vi "niFpga wdp fft input buffer.vi"(4 "enable":bool, 6 "write memory 2?":bool, 8 "read index":fxp<+,9,9>, 9 "write index":fxp<+,8,8>, 10 "data in im":fxp<+/-,8,1>[](array[numeric])=[0.0, 0.0], 11 "data in re":fxp<+/-,8,1>[](array[numeric])=[0.0, 0.0]) -> (2 "data out 1":T1, 3 "data out 0":T1)   [LabVIEW 2017]
uses:
  <vilib>/rvi/Analysis/measure/FFT/config/niFpgaFFTIOPattern.ctl
  <vilib>/rvi/Emulation/niFpgaSctlEmulationGetInTimedLoop.vi
  <vilib>/Utility/error.llb/Clear Errors.vi
  <vilib>/rvi/DataTransferAndStorage/Container/Common/niFpgaContainerGetUniqueNameForEmu.vi
  <vilib>/rvi/DataTransferAndStorage/Container/Common/niFpgaContainerSetEmuInfo.vi
  <vilib>/rvi/eio/common/nirviEmuReportErrorAndStop.vi
  <vilib>/rvi/DataTransferAndStorage/Container/Common/niFpgaContainerExecOnDevCompGetState.vi
  <vilib>/rvi/Emulation/niFpgaEmulationIsFPGAContextNoSignature.vi
  <vilib>/rvi/Emulation/niFpgaProcessEmulError.vi
  <vilib>/rvi/errors/nirviReportUnexpectedCaseInternalError (U32).vi
  <vilib>/rvi/Memory/Memory_Emulation/niFpgaMemoryEmulationCacheClearOnFirstRun.vi
  <vilib>/rvi/Memory/Memory_Emulation/nirvimemoryEmulationManagerCache_MakeExclusive.vi
  <vilib>/rvi/Memory/Memory_Emulation/niFpgaMemoryEmulationValidateCache.vi
  <vilib>/rvi/Memory/Memory_Emulation/nirvimemoryEmulationManagerCache_InsertValue.vi
  <vilib>/rvi/Memory/Memory_Emulation/nirvimemoryEmulationManagerCache_ReleaseExclusive.vi
  <vilib>/rvi/Memory/Memory_Emulation/nirvimemoryEmulationManagerCache_GetValue.vi
  <vilib>/rvi/Memory/Memory_Emulation/nirvimemoryEmulationManagerCache_SetValue.vi
  <vilib>/rvi/Emulation/niFpgaSctlEmulationResourceMgr.vi
  <vilib>/rvi/LocalResourceManager/LocalResourceManager.xnode
  <vilib>/rvi/DataTransferAndStorage/Container/XNode/niFpgaContainer.xnode
  <vilib>/rvi/Memory/Memory_Emulation/niFpgaMemoryEmulationRefIn.vi
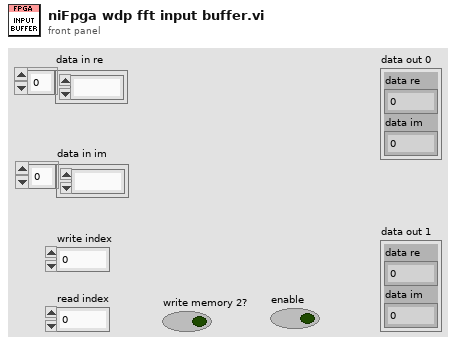
[diagram p1: front panel]
types:
  T1 = cluster{"internal input type":fxp<+/-,8,1>, "internal input type":fxp<+/-,8,1>}
  T2 = typedef "niFpgaFFTIOPattern.ctl" = enum16{"CI/CO", "CI/DO", "DI/CO"}
  T3 = cluster{"data":fxp<+/-,8,1>, "data":fxp<+/-,8,1>}
  T4 = cluster{"dara re":fxp<+/-,8,1>, "dara im":fxp<+/-,8,1>}
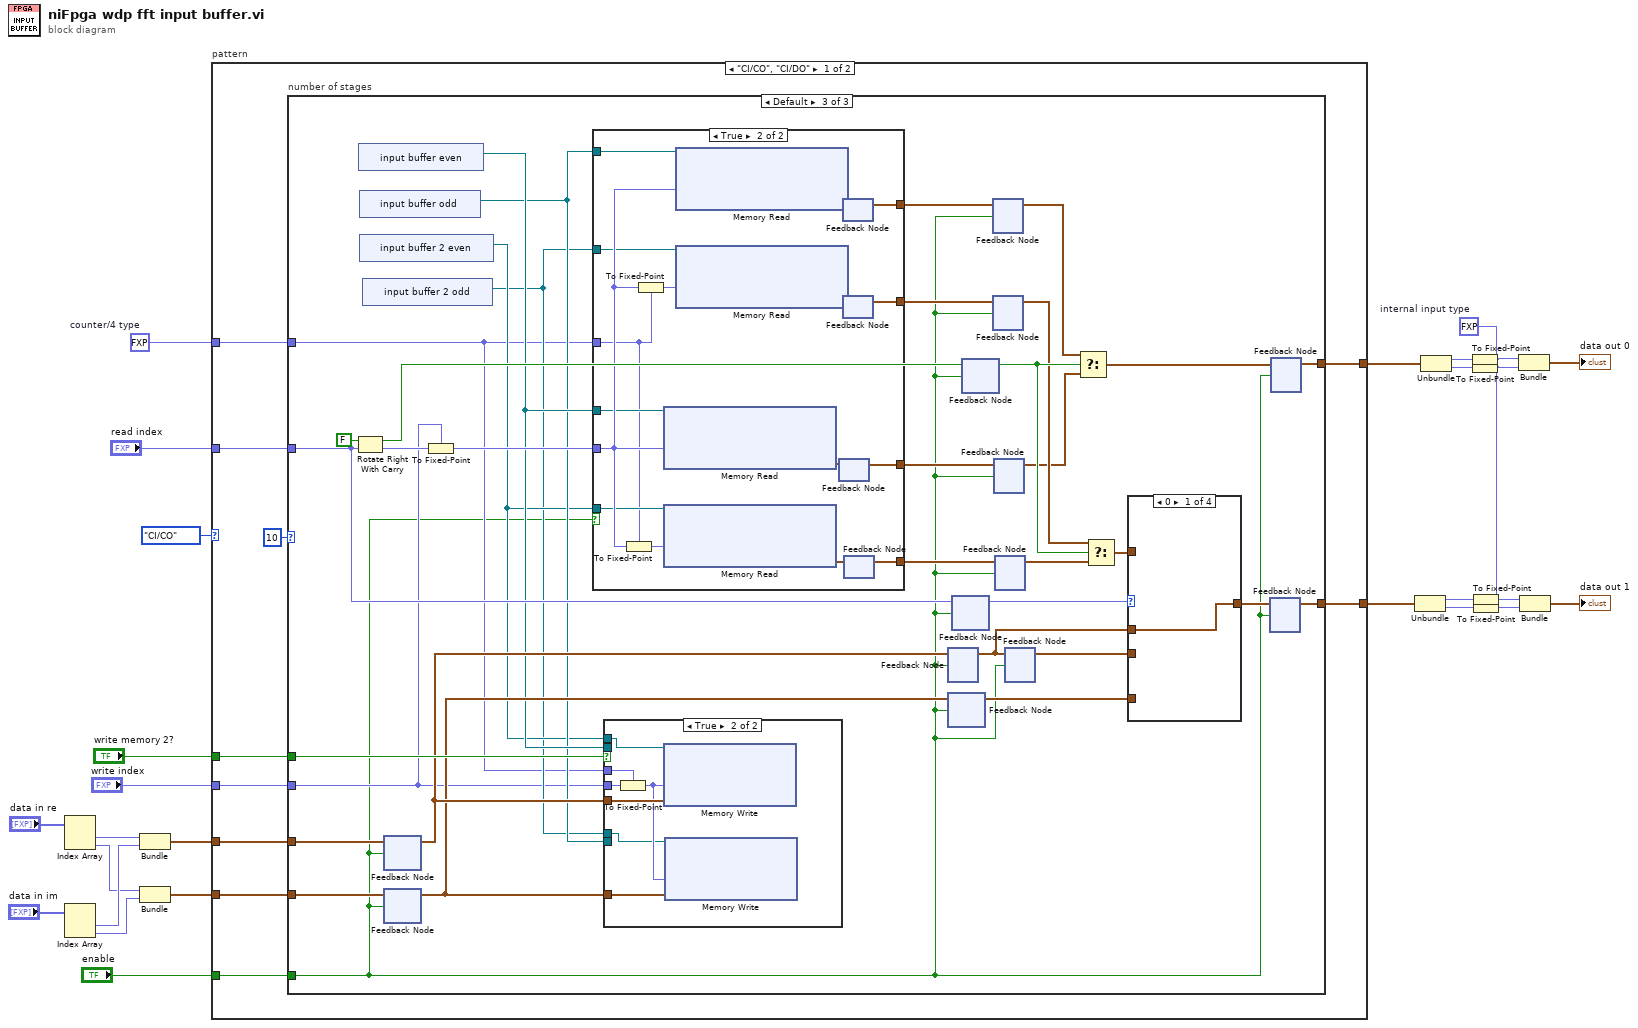
[diagram p0: block diagram]
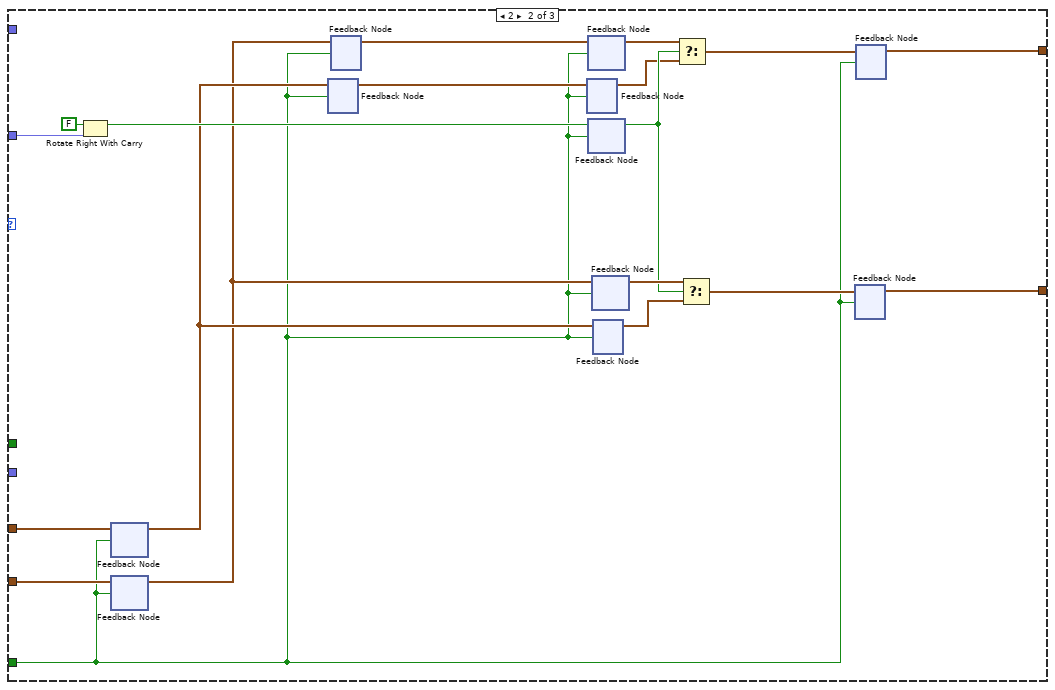
[diagram p3: hidden frame]
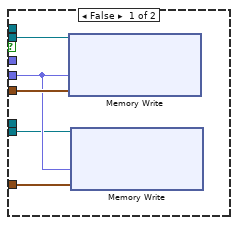
[diagram p8: hidden frame]
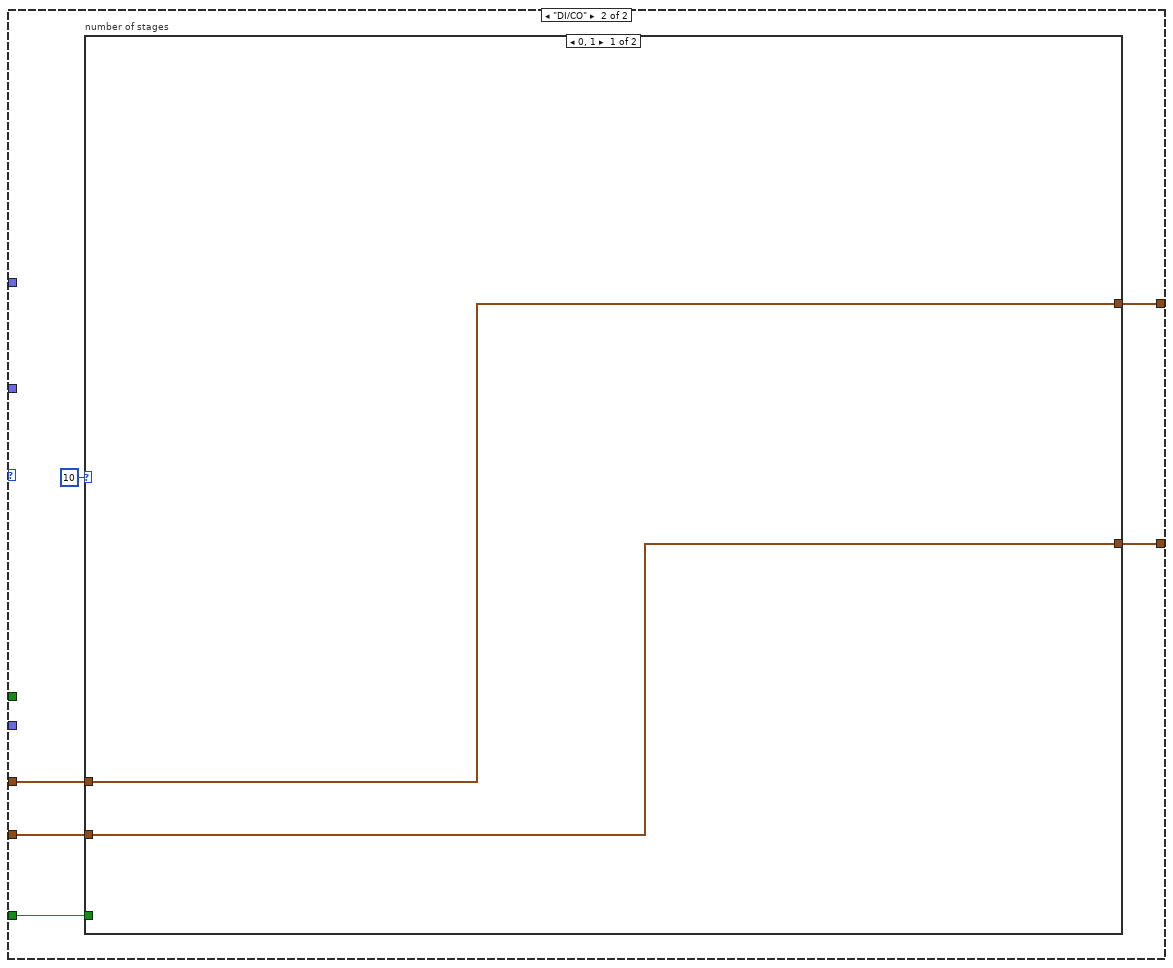
[diagram p9: hidden frame]
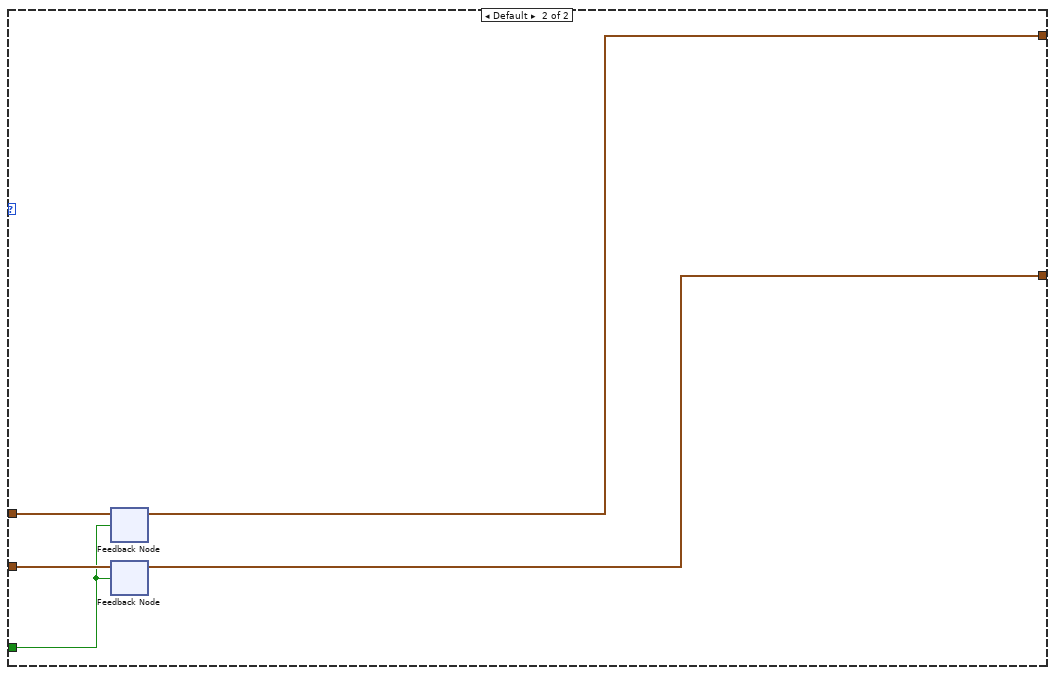
[diagram p10: hidden frame]
diagram:
  w1 = fxp<+,7,7> 0.0  # counter/4 type
  w18 = fxp<+/-,8,1> 0.0  # internal input type
  n1 = Index Array(array="data in re") -> (element #1=w10:fxp<+/-,8,1>, element #2=w8:fxp<+/-,8,1>)  [unwired: 2 in]
  n2 = Index Array(array="data in im") -> (element #1=w9:fxp<+/-,8,1>, element #2=w7:fxp<+/-,8,1>)  [unwired: 2 in]
  n3 = Bundle("data"=w10, "data"=w9) -> (w6:T3)  [unwired: 1 in]
  n4 = Bundle("data"=w8, "data"=w7) -> (w5:T3)  [unwired: 1 in]
  n5 = case "pattern" shown="\"CI/CO\", \"CI/DO\"" niFpgaFFTIOPattern."CI/CO" ("data in 0") {
    tunnel: "write index" -> [w37 _]
    tunnel: "read index" -> [w36 _]
    tunnel: "write memory 2?" -> [w34 _]
    tunnel: "enable" -> [w33 w130]
    tunnel: [w32 w129] -> w16
    tunnel: [w31 w128] -> w13
    tunnel: w6 -> [w30 w127]
    tunnel: w5 -> [w29 w126]
    tunnel: w1 -> [w28 _]
    frame "CI/CO", "CI/DO" {
      n6 = case "number of stages" shown="Default" u8 10 ("data in 0") {
        tunnel: w34 -> [_ _ w85]
        tunnel: w36 -> [_ w57 w84]
        tunnel: w33 -> [_ w40 w59]
        tunnel: w37 -> [_ _ w67]
        tunnel: w28 -> [_ _ w66]
        tunnel: [w39 w43 w62] -> w32
        tunnel: [w38 w41 w60] -> w31
        tunnel: w30 -> [w39 w46 w65]
        tunnel: w29 -> [w38 w45 w64]
        frame 0, 1 {
        }
        frame 2 {
          n7 = Rotate Right With Carry(2:w57, 3:FALSE ("carry")) -> (1:w56:bool)  [unwired: 1 out]
          n8 = feedback #1() -> (w52:T3)  [unwired: 1 out]
          n9 = feedback-in #1(w46, w40) -> ()
          n10 = feedback #2() -> (w51:T3)  [unwired: 1 out]
          n11 = feedback-in #2(w45, w40) -> ()
          n12 = feedback-in #3(w52, w40) -> ()
          n13 = feedback #3() -> (w50:T3)  [unwired: 1 in]
          n14 = feedback #4() -> (w48:T3)  [unwired: 1 in]
          n15 = feedback-in #4(w51, w40) -> ()
          n16 = feedback #5() -> (w49:T3)  [unwired: 1 in]
          n17 = feedback-in #5(w50, w40) -> ()
          n18 = feedback #6() -> (w47:T3)  [unwired: 1 in]
          n19 = feedback-in #6(w48, w40) -> ()
          n20 = feedback #7() -> (w53:bool)  [unwired: 1 out]
          n21 = feedback-in #7(w56, w40) -> ()
          n22 = feedback #8() -> (w55:T3)  [unwired: 1 out]
          n23 = feedback-in #8(w51, w40) -> ()
          n24 = feedback #9() -> (w54:T3)  [unwired: 1 out]
          n25 = feedback-in #9(w52, w40) -> ()
          n26 = Select(t=w47, s=w53, f=w49) -> (s? t:f=w44:T3)
          n27 = Select(t=w55, s=w53, f=w54) -> (s? t:f=w42:T3)
          n28 = feedback #10() -> (w41:T3)  [unwired: 1 in]
          n29 = feedback-in #10(w42, w40) -> ()
          n30 = feedback #11() -> (w43:T3)  [unwired: 1 in]
          n31 = feedback-in #11(w44, w40) -> ()
        }
        frame Default {
          n32 = Rotate Right With Carry(2:w84, 3:FALSE ("carry")) -> (0:w92:fxp<+,9,9>, 1:w88:bool)
          n33 = xnode "input buffer even"() -> ("Memory Out"=w71:refnum<k21>)
          n34 = xnode "input buffer odd"() -> ("Memory Out"=w70:refnum<k21>)
          n35 = xnode "input buffer 2 even"() -> ("Memory Out"=w69:refnum<k21>)
          n36 = xnode "input buffer 2 odd"() -> ("Memory Out"=w68:refnum<k21>)
          n37 = feedback #12() -> (w83:T3)  [unwired: 1 out]
          n38 = feedback-in #12(w65, w59) -> ()
          n39 = feedback #13() -> (w82:T3)  [unwired: 1 out]
          n40 = feedback-in #13(w64, w59) -> ()
          n41 = To Fixed-Point(fixed-point type=w67, number=w92) -> (fixed-point=w89:fxp<+,8,8>)
          n42 = case shown="True" w59 {
            tunnel: w89 -> [_ w103]
            tunnel: [_ w102] -> w81
            tunnel: [_ w101] -> w79
            tunnel: [_ w100] -> w77
            tunnel: [_ w99] -> w75
            tunnel: w70 -> [_ w98]
            tunnel: w68 -> [_ w97]
            tunnel: w71 -> [_ w96]
            tunnel: w69 -> [_ w95]
            tunnel: w66 -> [_ w94]
            frame False {
            }
            frame True {
              n43 = To Fixed-Point(fixed-point type=w94, number=w103) -> (fixed-point=w106:fxp<+,7,7>)
              n44 = To Fixed-Point(fixed-point type=w94, number=w103) -> (fixed-point=w107:fxp<+,7,7>)
              n45 = xnode ("Memory Read")("Address"=w103, "Memory In"=w96) -> ("Data"=w105:T4)  [unwired: 1 out]
              n46 = xnode ("Memory Read")("Address"=w106, "Memory In"=w95) -> ("Data"=w104:T4)  [unwired: 1 out]
              n47 = xnode ("Memory Read")("Address"=w103, "Memory In"=w98) -> ("Data"=w109:T4)  [unwired: 1 out]
              n48 = xnode ("Memory Read")("Address"=w107, "Memory In"=w97) -> ("Data"=w108:T4)  [unwired: 1 out]
              n49 = feedback #14() -> (w100:T4)  [unwired: 1 out]
              n50 = feedback-in #14(w105) -> ()
              n51 = feedback #15() -> (w102:T4)  [unwired: 1 out]
              n52 = feedback-in #15(w109) -> ()
              n53 = feedback #16() -> (w101:T4)  [unwired: 1 out]
              n54 = feedback-in #16(w108) -> ()
              n55 = feedback #17() -> (w99:T4)  [unwired: 1 out]
              n56 = feedback-in #17(w104) -> ()
            }
          }
          n57 = case shown="True" w85 {
            tunnel: w83 -> [w118 w125]
            tunnel: w67 -> [w116 w124]
            tunnel: w82 -> [w117 w122]
            tunnel: w71 -> [w115 _]
            tunnel: w70 -> [w114 _]
            tunnel: w69 -> [_ w121]
            tunnel: w68 -> [_ w120]
            tunnel: w66 -> [_ w119]
            frame False {
              n58 = xnode ("Memory Write")("Address"=w116, "Data"=w118, "Memory In"=w115) -> ()  [unwired: 1 out]
              n59 = xnode ("Memory Write")("Address"=w116, "Data"=w117, "Memory In"=w114) -> ()  [unwired: 1 out]
            }
            frame True {
              n60 = To Fixed-Point(fixed-point type=w119, number=w124) -> (fixed-point=w123:fxp<+,7,7>)
              n61 = xnode ("Memory Write")("Address"=w123, "Data"=w125, "Memory In"=w121) -> ()  [unwired: 1 out]
              n62 = xnode ("Memory Write")("Address"=w123, "Data"=w122, "Memory In"=w120) -> ()  [unwired: 1 out]
            }
          }
          n63 = feedback #18() -> (w72:T3)  [unwired: 1 out]
          n64 = feedback-in #18(w83, w59) -> ()
          n65 = feedback #19() -> (w90:T3)  [unwired: 1 out]
          n66 = feedback-in #19(w82, w59) -> ()
          n67 = feedback #20() -> (w91:fxp<+,9,9>)  [unwired: 1 out]
          n68 = feedback-in #20(w84, w59) -> ()
          n69 = feedback #21() -> (w87:bool)  [unwired: 1 out]
          n70 = feedback-in #21(w88, w59) -> ()
          n71 = feedback #22() -> (w80:T4)  [unwired: 1 out]
          n72 = feedback-in #22(w81, w59) -> ()
          n73 = feedback #23() -> (w78:T4)  [unwired: 1 out]
          n74 = feedback-in #23(w79, w59) -> ()
          n75 = feedback #24() -> (w76:T4)  [unwired: 1 out]
          n76 = feedback-in #24(w77, w59) -> ()
          n77 = feedback #25() -> (w74:T4)  [unwired: 1 out]
          n78 = feedback-in #25(w75, w59) -> ()
          n79 = feedback #26() -> (w73:T3)  [unwired: 1 out]
          n80 = feedback-in #26(w72, w59) -> ()
          n81 = Select(t=w80, s=w87, f=w76) -> (s? t:f=w63:T4)
          n82 = Select(t=w78, s=w87, f=w74) -> (s? t:f=w86:T4)
          n83 = case shown="0" w91 {
            tunnel: [w110 w111 w112 w113] -> w61
            tunnel: w73 -> [_ _ w112 _]
            tunnel: w72 -> [w110 _ _ _]
            tunnel: w90 -> [_ w111 _ _]
            tunnel: w86 -> [_ _ _ w113]
            frame 0 {
            }
            frame 1 {
            }
            frame 2 {
            }
            frame Default {
            }
          }
          n84 = feedback #27() -> (w60:T4)  [unwired: 1 in]
          n85 = feedback-in #27(w61, w59) -> ()
          n86 = feedback #28() -> (w62:T4)  [unwired: 1 in]
          n87 = feedback-in #28(w63, w59) -> ()
        }
      }
    }
    frame "DI/CO" {
      n88 = case "number of stages" shown="0, 1" u8 10 ("data in 0") {
        tunnel: w130 -> [_ w136]
        tunnel: [w133 w135] -> w129
        tunnel: [w132 w134] -> w128
        tunnel: w127 -> [w133 w138]
        tunnel: w126 -> [w132 w137]
        frame 0, 1 {
        }
        frame Default {
          n89 = feedback #29() -> (w135:T3)  [unwired: 1 out]
          n90 = feedback-in #29(w138, w136) -> ()
          n91 = feedback #30() -> (w134:T3)  [unwired: 1 out]
          n92 = feedback-in #30(w137, w136) -> ()
        }
      }
    }
  }
  n93 = Unbundle(w13) -> ("data"=w12:fxp<+/-,8,1>, "data"=w11:fxp<+/-,8,1>)
  n94 = Unbundle(w16) -> ("data"=w15:fxp<+/-,8,1>, "data"=w14:fxp<+/-,8,1>)
  n95 = To Fixed-Point(fixed-point type=w18, number=w15) -> (fixed-point=w19:fxp<+/-,8,1>)
  n96 = To Fixed-Point(fixed-point type=w18, number=w14) -> (fixed-point=w20:fxp<+/-,8,1>)
  n97 = To Fixed-Point(fixed-point type=w18, number=w12) -> (fixed-point=w21:fxp<+/-,8,1>)
  n98 = To Fixed-Point(fixed-point type=w18, number=w11) -> (fixed-point=w22:fxp<+/-,8,1>)
  n99 = Bundle("internal input type"=w19, "internal input type"=w20) -> (→"data out 0":T1)  [unwired: 1 in]
  n100 = Bundle("internal input type"=w21, "internal input type"=w22) -> (→"data out 1":T1)  [unwired: 1 in]
